vi "Reference_new version_1.0.vi"(1 "Phase log in":dbl=0.9999999999996251, 2 "AI Block Size":i32=40000, 4 "Phase&time":T1, 5 "Reset":bool, 6 "Frequency":dbl=20.0 format="%.2f", 7 "Ref Shape":enum16{"Sine", "Square"}(ring), 8 "Ref Amp":dbl=5.0 format="%.2f", 9 "AI Rate":dbl=200000.0) -> (0 "Ref out":T2={"Ref X"=array[40000 elements], "Ref Y"=array[40000 elements], "AI Rate"=200000.0, "AI Block Size"=40000.0, "Frequency"=20.0, "Ref amp"=5.0} {"Ref amp" step=0.001 format="%0.4f"; "Frequency" step=0.001 format="%0.4f"; "AI Block Size" step=0.001 format="%0.4f"; "AI Rate" step=0.001 format="%0.4f"}, 3 "Phase log":dbl=0.9999999999996251)   [LabVIEW 2011, in "Lock-In Variable Channels_2.lvclass"]
uses:
  Variable Channel O.O.P/Lock-In Variable Channels_2.lvclass
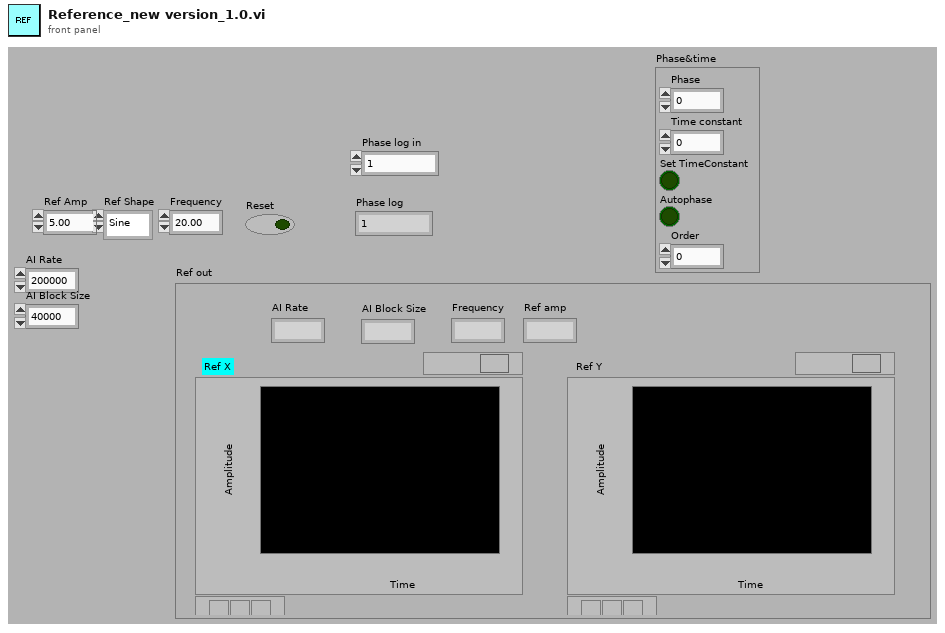
[diagram p1: front panel]
types:
  T1 = cluster{"Phase":dbl, "Time constant":dbl, "Set TimeConstant":bool, "Autophase":bool, "Order":dbl}
  T2 = cluster{"Ref X":dbl[], "Ref Y":dbl[], "AI Rate":dbl, "AI Block Size":dbl, "Frequency":dbl, "Ref amp":dbl}
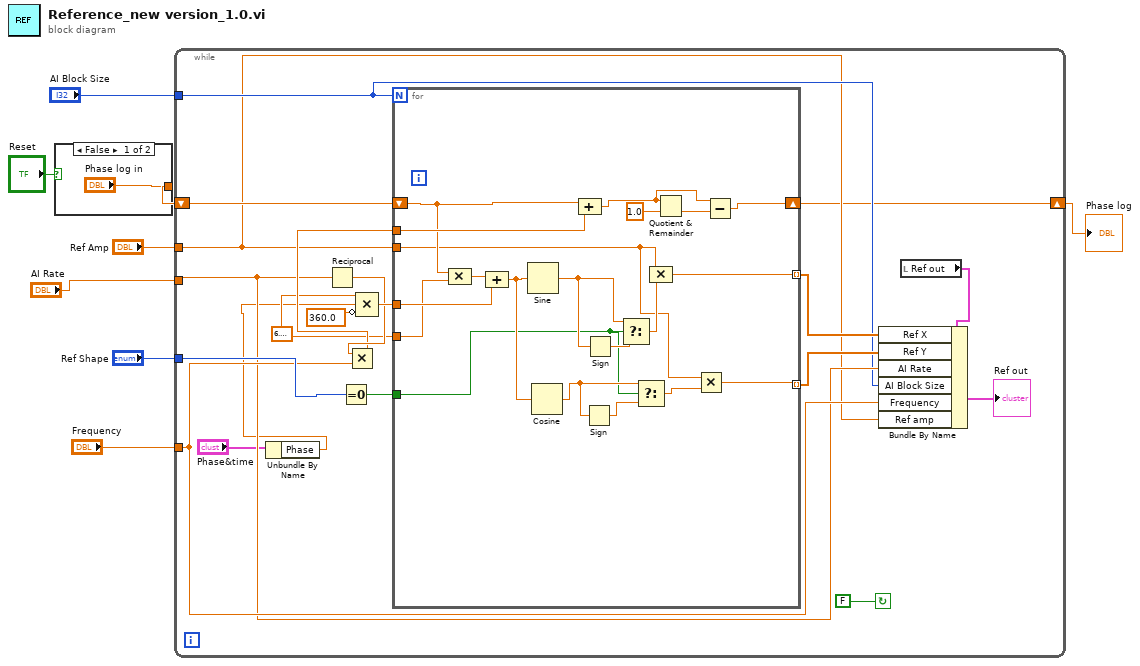
[diagram p0: block diagram]
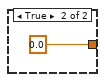
[diagram p2: hidden frame]
diagram:
  n1 = case shown="False" "Reset" {
    tunnel: ["Phase log in" 0.0] -> w5
    frame False {
    }
    frame True {
    }
  }
  n2 = while {
    shift-left: w5 -> [w30]
    shift-right: [w11] -> w3
    tunnel: "AI Block Size" -> [w17]
    tunnel: "Ref Amp" -> [w16]
    tunnel: "AI Rate" -> [w18]
    tunnel: "Ref Shape" -> [w25]
    tunnel: "Frequency" -> [w19]
    stop <- FALSE continue-if-true
    w22 = 6.283185307179586
    n3 = Unbundle By Name("Phase&time") -> ("Phase"=w12:dbl)
    n4 = Reciprocal(x=w18) -> (1/x=w24:dbl)
    n5 = Equal To 0?(x=w25) -> (x = 0?=w28:bool)
    n6 = Multiply(x=w24, y=w19) -> (x*y=w23:dbl)
    n7 = Compound Arithmetic op=MULTIPLY(w12, w22, invert 360.0 ("value")) -> (w27:dbl)
    n8 = for {
      N: w17 -> [_]
      shift-right: [w39] -> w11
      shift-left: w30 -> [w44]
      tunnel: w23 -> [w50]
      tunnel: w16 -> [w32]
      tunnel: w28 -> [w34]
      tunnel: w27 -> [w47]
      tunnel: [w43] -> w21 mode=indexing
      tunnel: w22 -> [w38]
      tunnel: [w31] -> w20 mode=indexing
      n9 = Compound Arithmetic op=MULTIPLY(w44, w38) -> (w48:dbl)
      n10 = Compound Arithmetic op=ADD(w48, w47) -> (w37:dbl)
      n11 = Sine(x=w37) -> (sin(x)=w46:dbl)
      n12 = Cosine(x=w37) -> (cos(x)=w36:dbl)
      n13 = Compound Arithmetic op=ADD(w44, w50) -> (w41:dbl)
      n14 = Sign(1:w36) -> (0:w35:dbl)
      n15 = Sign(1:w46) -> (0:w45:dbl)
      n16 = Select(t=w46, s=w34, f=w45) -> (s? t:f=w49:dbl)
      n17 = Select(t=w36, s=w34, f=w35) -> (s? t:f=w33:dbl)
      n18 = Compound Arithmetic op=MULTIPLY(w32, w49) -> (w43:dbl)
      n19 = Quotient & Remainder(x=w41, y=1.0) -> (floor(x/y)=w40:dbl)  [unwired: 1 out]
      n20 = Multiply(x=w32, y=w33) -> (x*y=w31:dbl)
      n21 = Subtract(x=w41, y=w40) -> (x-y=w39:dbl)
    }
    n22 = local read "Ref out"() -> (w15:T2)
    n23 = Bundle By Name(cluster=w15, "Ref X"=w21, "Ref Y"=w20, "AI Rate"=w18, "AI Block Size"=w17, "Frequency"=w19, "Ref amp"=w16) -> (→"Ref out":T2)
  }
  "Phase log" <- w3
